vi "rethinkdb_hashlib_hexlify.vi"(11 "sha256":u32[](array[numeric]) format="%08x") -> (3 "hex (0-9a-f)":string)   [LabVIEW 2017]
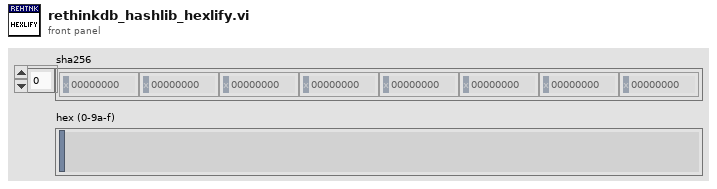
[diagram p1: front panel]
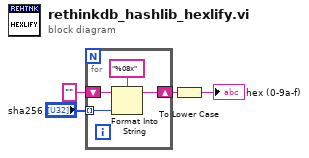
[diagram p0: block diagram]
diagram:
  n1 = for {
    tunnel: "sha256" -> [w8] mode=indexing
    shift-right: [w7] -> w2
    shift-left: "" -> [w6]
    n2 = Format Into String(format string="%08x", initial string=w6, w8) -> (resulting string=w7:string)  [unwired: 1 in, 1 out]
  }
  n3 = To Lower Case(string=w2) -> (all lower case string=→"hex (0-9a-f)":string)
